vi "oax_Get Waveform Subset.vi"(4 "duration":dbl, 6 "start index":dbl, 8 "error in (no error)":errorcluster, 9 "Tach Signal":waveform(dbl), 10 "Vibration Signal Y":waveform(dbl), 11 "Vibration Signal X":waveform(dbl)) -> (0 "error out":errorcluster, 1 "Tach Signal out":waveform(dbl), 2 "Vibration Signal Y out":waveform(dbl), 3 "Vibration Signal X out":waveform(dbl))   [LabVIEW 2017]
uses:
  <vilib>/Waveform/WDTOps.llb/WDT Get Waveform Subset DBL (LV80).vi
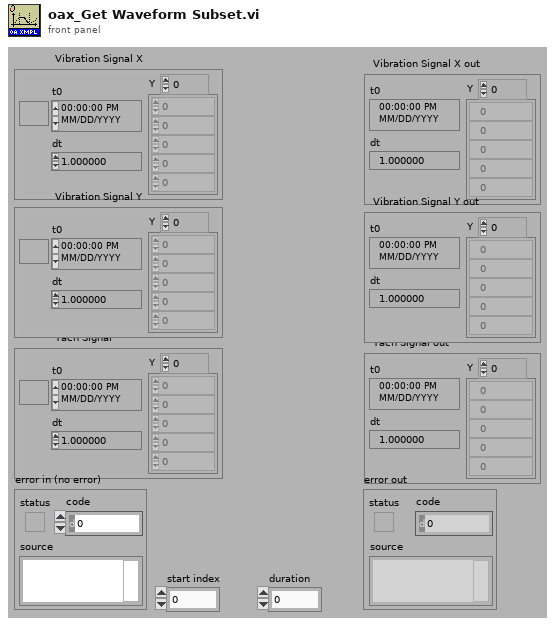
[diagram p1: front panel]
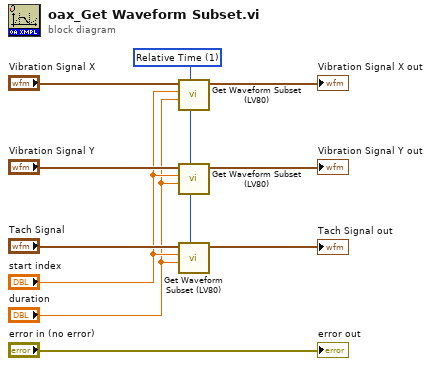
[diagram p0: block diagram]
diagram:
  w1 = u16 1 items=["Index", "Relative Time"] ("Mode")
  n1 = call-poly <vilib>:"Get Waveform Subset (LV80).vi"("start/duration format"=w1, "duration"="duration", "start samples/time"="start index", "waveform in"="Vibration Signal X") -> ("waveform out"=→"Vibration Signal X out":waveform(dbl))  [unwired: 2 in, 3 out]
  n2 = call-poly <vilib>:"Get Waveform Subset (LV80).vi"("start/duration format"=w1, "duration"="duration", "start samples/time"="start index", "waveform in"="Vibration Signal Y") -> ("waveform out"=→"Vibration Signal Y out":waveform(dbl))  [unwired: 2 in, 3 out]
  n3 = call-poly <vilib>:"Get Waveform Subset (LV80).vi"("start/duration format"=w1, "duration"="duration", "start samples/time"="start index", "waveform in"="Tach Signal") -> ("waveform out"=→"Tach Signal out":waveform(dbl))  [unwired: 2 in, 3 out]
  "error out" <- "error in (no error)"
